vi "FRCts20_EspEngine_ConverToEvent.vi"(8 "error in (no error)":errorcluster, 10 "Single Event":T2) -> (0 "error out":errorcluster, 2 "Event":T4)   [LabVIEW 2014, in "FRCts20_EspEngine.lvlib"]
uses:
  FRCts20_EspEngine.lvlib
  TypeDefs/FRCts20_EspEngine_Event.ctl
  Web Methods/source/VI Source/Web Method Public Interface/FRCts20_WebMethods_ctl_singleEvent.ctl
  Web Methods/source/VI Source/Web Method Public Interface/FRCts20_WebMethods_ctl_teamIdentifier.ctl
  Web Methods/source/VI Source/FRCts20_WebMethods.lvlib
panel:
  in  "Requests":T1(array[cluster])=[{"RequestId"=1, "Request Description"="this is my next", "Team Number"=44}, {"RequestId"=2, "Request Description"="request description", "Team Number"=66}, {"RequestId"=3, "Request Description"="lolz w-hat", "Team Number"=77}]
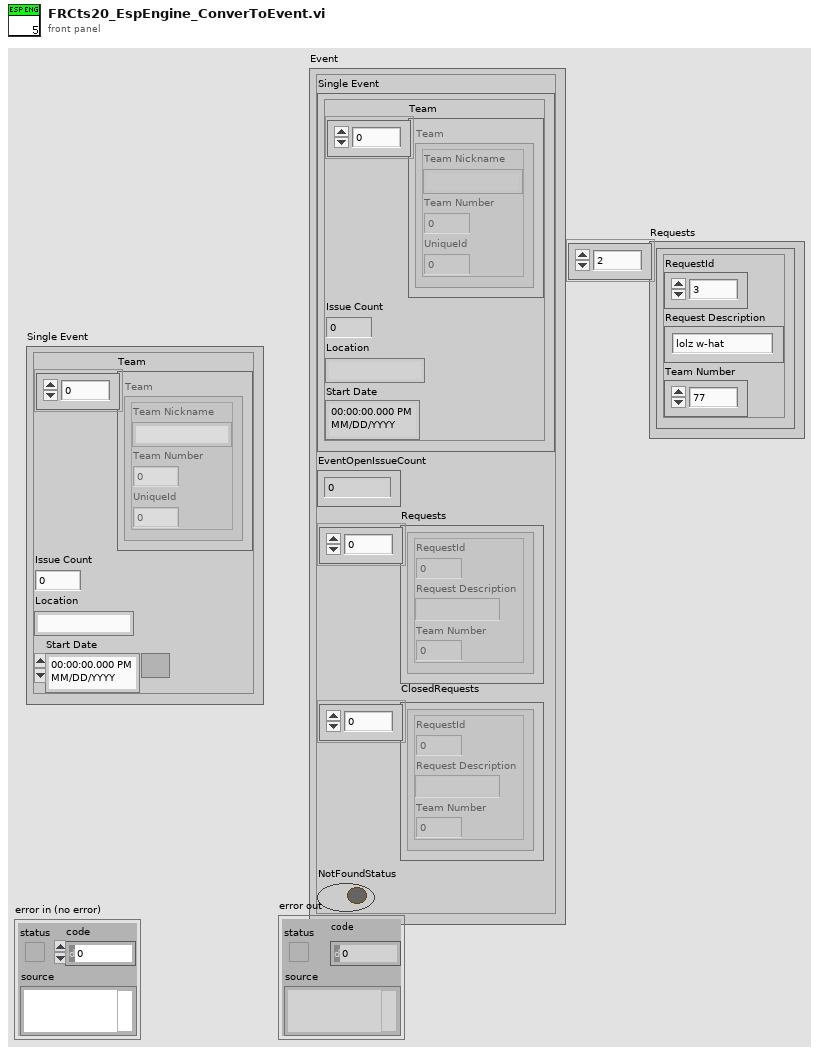
[diagram p1: front panel]
types:
  T1 = cluster{"RequestId":i32, "Request Description":string, "Team Number":i32}[]
  T2 = typedef "FRCts20_WebMethods.lvlib/FRCts20_WebMethods_ctl_singleEvent.ctl" = cluster{"Team":T3[], "Issue Count":i32, "Location":string, "Start Date ":timestamp}
  T3 = typedef "FRCts20_WebMethods.lvlib/FRCts20_WebMethods_ctl_teamIdentifier.ctl" = cluster{"Team Nickname":string, "Team Number ":u32, "UniqueId":u32}
  T4 = typedef "FRCts20_EspEngine.lvlib/FRCts20_EspEngine_Event.ctl" = cluster{"Single Event":T2, "EventOpenIssueCount":i16, "Requests":cluster{"RequestId":i32, "Request Description":string, "Team Number":i32}[], "ClosedRequests":cluster{"RequestId":i32, "Request Description":string, "Team Number":i32}[], "NotFoundStatus":bool}
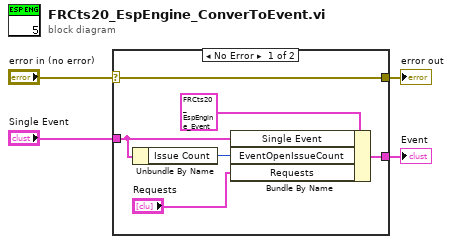
[diagram p0: block diagram]
diagram:
  n1 = case shown="No Error" "error in (no error)" {
    selector: "error in (no error)" -> [w6 w11]
    tunnel: [w6 w11] -> w4
    tunnel: "Single Event" -> [w9 _]
    tunnel: [w7 _] -> w1
    frame No Error {
      n2 = Unbundle By Name(w9) -> ("Issue Count"=w10:i32)
      n3 = Bundle By Name(cluster=T4 {"Single Event"={"Team"=[], "Issue Count"=0, "Location"="", "Start Date "=timestamp(0 s since 1904-01-01)}, "EventOpenIssueCount"=0, "Requests"=[], "ClosedRequests"=[], "NotFoundStatus"=FALSE} ("Event"), "Single Event"=w9, "EventOpenIssueCount"=w10, "Requests"="Requests") -> (w7:T4)
    }
    frame Error {
    }
  }
  "Event" <- w1
  "error out" <- w4
